vi "NeglectedDetector.vi"(8 "error in (no error)":errorcluster, 9 "Days until Neglected":i16, 10 "SR Status":string, 11 "LastModified":timestamp) -> (0 "error out":errorcluster, 3 "Neglected":bool)   [LabVIEW 2018, in "Controller.lvlib"]
uses:
  Controller.lvlib
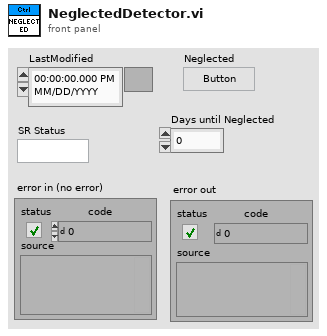
[diagram p1: front panel]
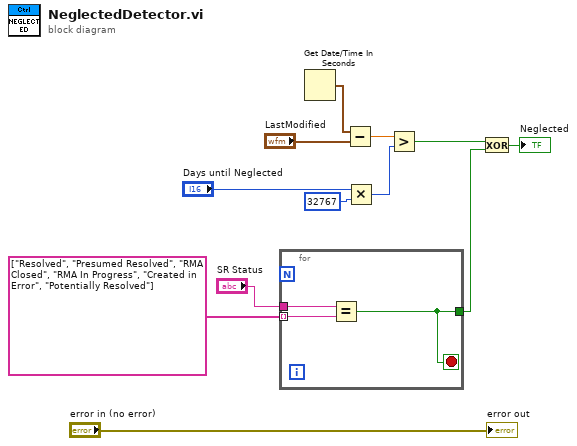
[diagram p0: block diagram]
diagram:
  n1 = for {
    tunnel: "SR Status" -> [w15]
    tunnel: [w14] -> w2
    tunnel: string[] ["Resolved", "Presumed Resolved", "RMA Closed", "RMA In Progress", "Created in Error", "Potentially Resolved"] -> [w13] mode=indexing
    stop <- w14 stop-if-true
    n2 = Equal?(x=w15, y=w13) -> (x = y?=w14:bool)
  }
  n3 = Get Date/Time In Seconds() -> (seconds since 1Jan1904=w12:timestamp)
  n4 = Subtract(x=w12, y="LastModified") -> (x-y=w9:dbl)
  n5 = Multiply(x="Days until Neglected", y=i16 32767) -> (x*y=w5:i16)
  n6 = Greater?(x=w9, y=w5) -> (0:w4:bool)
  n7 = Exclusive Or(1:w2, 2:w4) -> (0:→"Neglected":bool)
  "error out" <- "error in (no error)"
